vi "Race Conditions.vi"() -> ()   [LabVIEW 2020]
uses:
  FGV Map/Controls/FGV Map Core State.ctl
  FGV Map.lvlib
panel:
  out "Instance Out":map{string, variant}(c390)
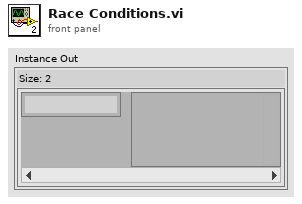
[diagram p1: front panel]
types:
  T1 = typedef "FGV Map.lvlib/FGV Map Core State.ctl" = enum16{"Init", "Set Instance (Unlock)", "Get Instance", "Get Instance (Lock)", "Unlock", "Get All Instances", "Delete Instance"}
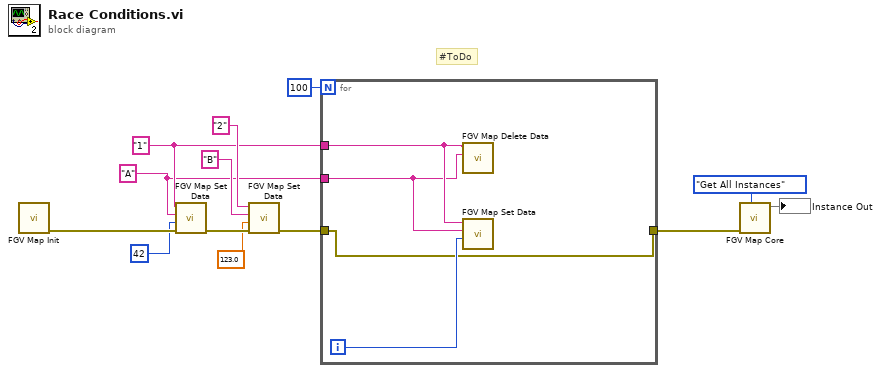
[diagram p0: block diagram]
diagram:
  w5 = "A" ("Data Key")
  w6 = "1" ("Instance Key")
  # "#ToDo"
  n1 = call "FGV Map Init.vi"() -> ("error out"=w13:errorcluster)  [unwired: 11 in]
  n2 = call "FGV Map Set Data.vi"("error in (no error)"=w13, "Data In"=42, "Data Key"=w5, "Instance Key"=w6) -> ("error out"=w11:errorcluster)  [unwired: 5 in, 2 out]
  n3 = call "FGV Map Set Data.vi"("error in (no error)"=w11, "Data In"=123.0, "Data Key"="B", "Instance Key"="2") -> ("error out"=w7:errorcluster)  [unwired: 5 in, 2 out]
  n4 = for {
    N: 100 -> [_]
    tunnel: w7 -> [w14]
    tunnel: w6 -> [w16]
    tunnel: w5 -> [w15]
    tunnel: [w14] -> w4
    i -> [w17]
    n5 = call "FGV Map Delete Data.vi"("Data Key"=w15, "Instance Key"=w16) -> ()  [unwired: 7 in, 3 out]
    n6 = call "FGV Map Set Data.vi"("Data In"=w17, "Data Key"=w15, "Instance Key"=w16) -> ()  [unwired: 6 in, 3 out]
  }
  n7 = call "FGV Map Core.vi"("FGV State"=FGV_Map_Core_State."Get All Instances", "error in"=w4) -> ("Instance Out"=→"Instance Out":map{string, variant})  [unwired: 5 in, 4 out]
